vi "2526 Open Ref.vi"(8 "error in":errorcluster, 11 "JSONCluster":T1) -> (0 "error out":errorcluster, 3 "IVI Refnum out":refnum<k15>)   [LabVIEW 2019, in "SupportVIs.lvlib"]
uses:
  SupportVIs.lvlib
  JSONCluster.ctl
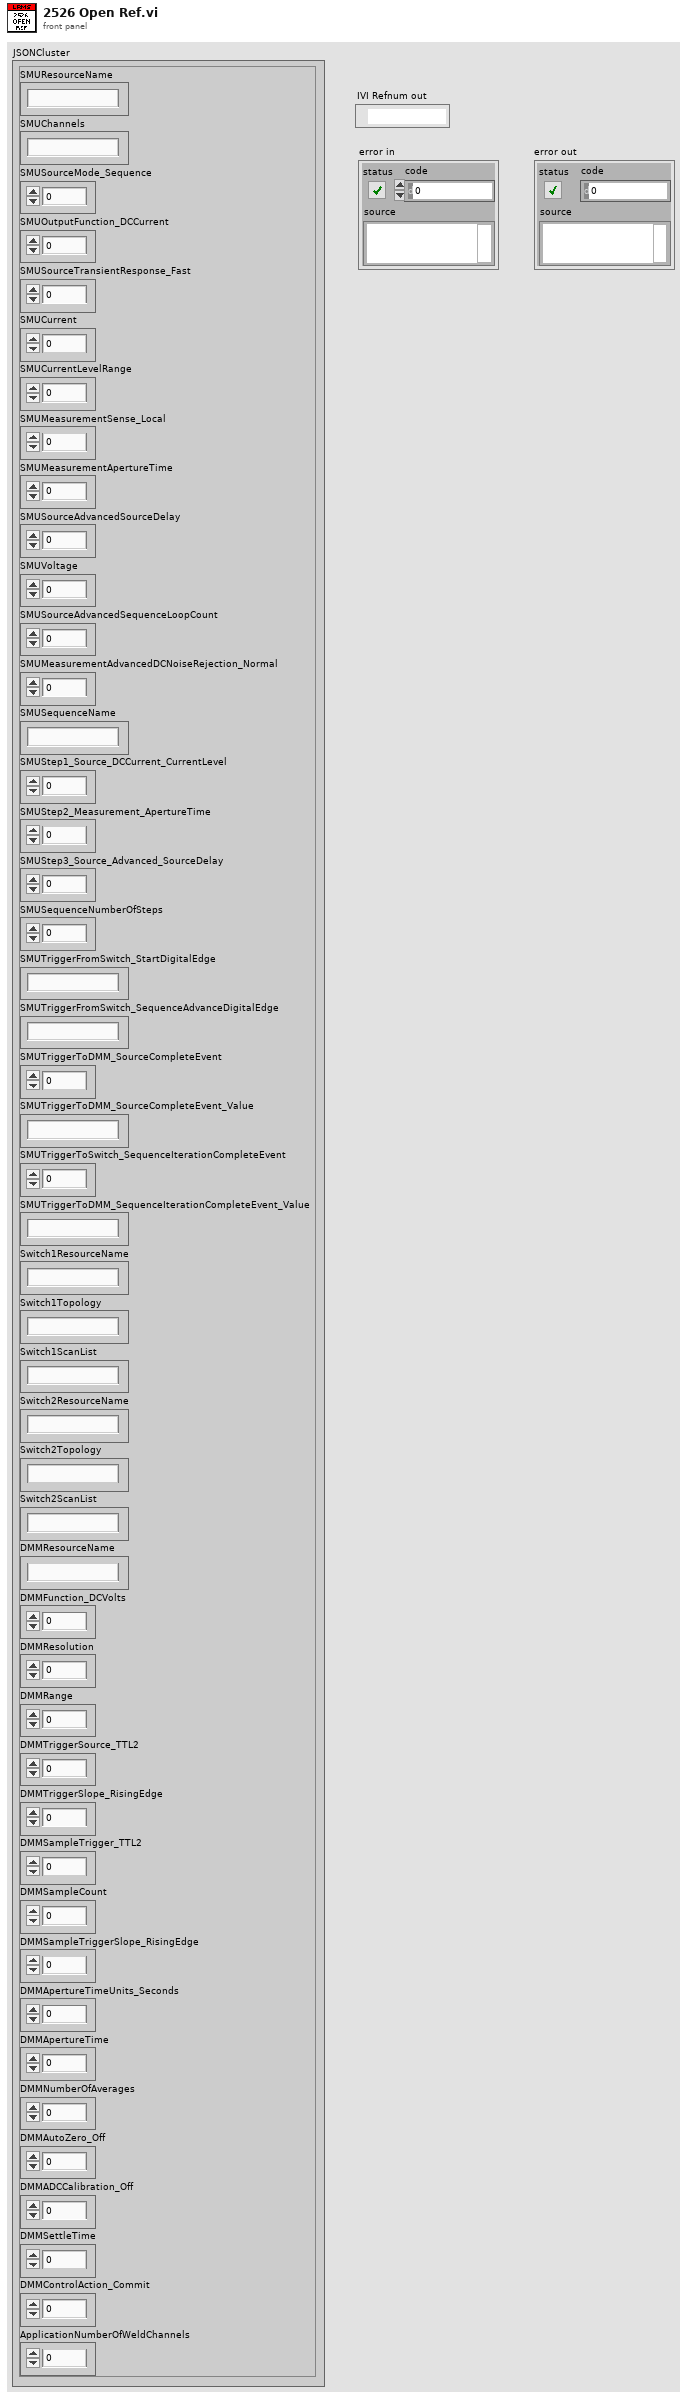
[diagram p1: front panel]
types:
  T1 = typedef "JSONCluster.ctl" = cluster{"SMUResourceName":string, "SMUChannels":string, "SMUSourceMode_Sequence":i32, "SMUOutputFunction_DCCurrent":i32, "SMUSourceTransientResponse_Fast":i32, "SMUCurrent":dbl, "SMUCurrentLevelRange":dbl, "SMUMeasurementSense_Local":i32, "SMUMeasurementApertureTime":dbl, "SMUSourceAdvancedSourceDelay":dbl, "SMUVoltage":dbl, "SMUSourceAdvancedSequenceLoopCount":i32, "SMUMeasurementAdvancedDCNoiseRejection_Normal":i32, "SMUSequenceName":string, "SMUStep1_Source_DCCurrent_CurrentLevel":i32, "SMUStep2_Measurement_ApertureTime":i32, "SMUStep3_Source_Advanced_SourceDelay":i32, "SMUSequenceNumberOfSteps":i32, "SMUTriggerFromSwitch_StartDigitalEdge":string, "SMUTriggerFromSwitch_SequenceAdvanceDigitalEdge":string, "SMUTriggerToDMM_SourceCompleteEvent":i32, "SMUTriggerToDMM_SourceCompleteEvent_Value":string, "SMUTriggerToSwitch_SequenceIterationCompleteEvent":i32, "SMUTriggerToDMM_SequenceIterationCompleteEvent_Value":string, "Switch1ResourceName":string, "Switch1Topology":string, "Switch1ScanList":string, "Switch2ResourceName":string, "Switch2Topology":string, "Switch2ScanList":string, "DMMResourceName":string, "DMMFunction_DCVolts":i32, "DMMResolution":dbl, "DMMRange":dbl, "DMMTriggerSource_TTL2":i32, "DMMTriggerSlope_RisingEdge":i32, "DMMSampleTrigger_TTL2":i32, "DMMSampleCount":i32, "DMMSampleTriggerSlope_RisingEdge":i32, "DMMApertureTimeUnits_Seconds":i32, "DMMApertureTime":dbl, "DMMNumberOfAverages":i32, "DMMAutoZero_Off":i32, "DMMADCCalibration_Off":i32, "DMMSettleTime":dbl, "DMMControlAction_Commit":i32, "ApplicationNumberOfWeldChannels":i32}
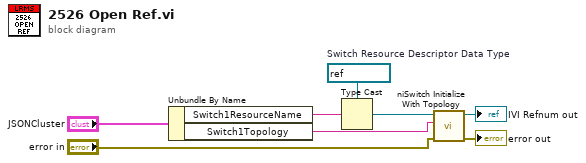
[diagram p0: block diagram]
diagram:
  w4 = refnum<k15> "2526_1"  # Switch Resource Descriptor Data Type
  n1 = Unbundle By Name("JSONCluster") -> ("Switch1ResourceName"=w5:string, "Switch1Topology"=w2:string)
  n2 = Type Cast(type=w4, x=w5) -> (*(type *) &x=w3:refnum<k15>)
  n3 = call <instrlib>:"niSwitch Initialize With Topology.vi"("error in (no error)"="error in", "topology name"=w2, "resource name"=w3) -> ("error out"=→"error out":errorcluster, "instrument handle out"=→"IVI Refnum out":refnum<k15>)  [unwired: 2 in, 5 out]
